vi "OS_Comm_to_Var_Binary.vi"(9 "Array 3":T1[](array[typedef]) {"Control" items=["Nul"=0, "Pulse On"=1, "Pulse Off"=2, "Latch On"=3, "Latch Off"=4, "Close"=65, "Trip"=129]}) -> ()   [LabVIEW 2016, in "DNP3_Outstation_Template.lvlib"]
uses:
  DNP3_Outstation_Template.lvlib
  <vilib>/DNP3/DNP3_Common/crob.ctl
  <vilib>/DNP3/DNP3_Common/crob_ctrl.ctl
  <vilib>/Utility/file.llb/Read Delimited Spreadsheet (string).vi
  <vilib>/DNP3/DNP3_Common.lvlib
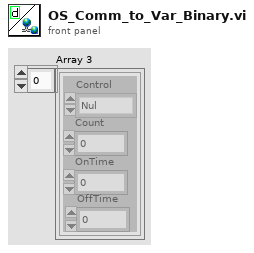
[diagram p1: front panel]
types:
  T1 = typedef "DNP3_Common.lvlib/crob.ctl" = cluster{"OnTime":u32, "Count":u8, "OffTime":u32, "Control":T2}
  T2 = typedef "DNP3_Common.lvlib/crob_ctrl.ctl" = u8
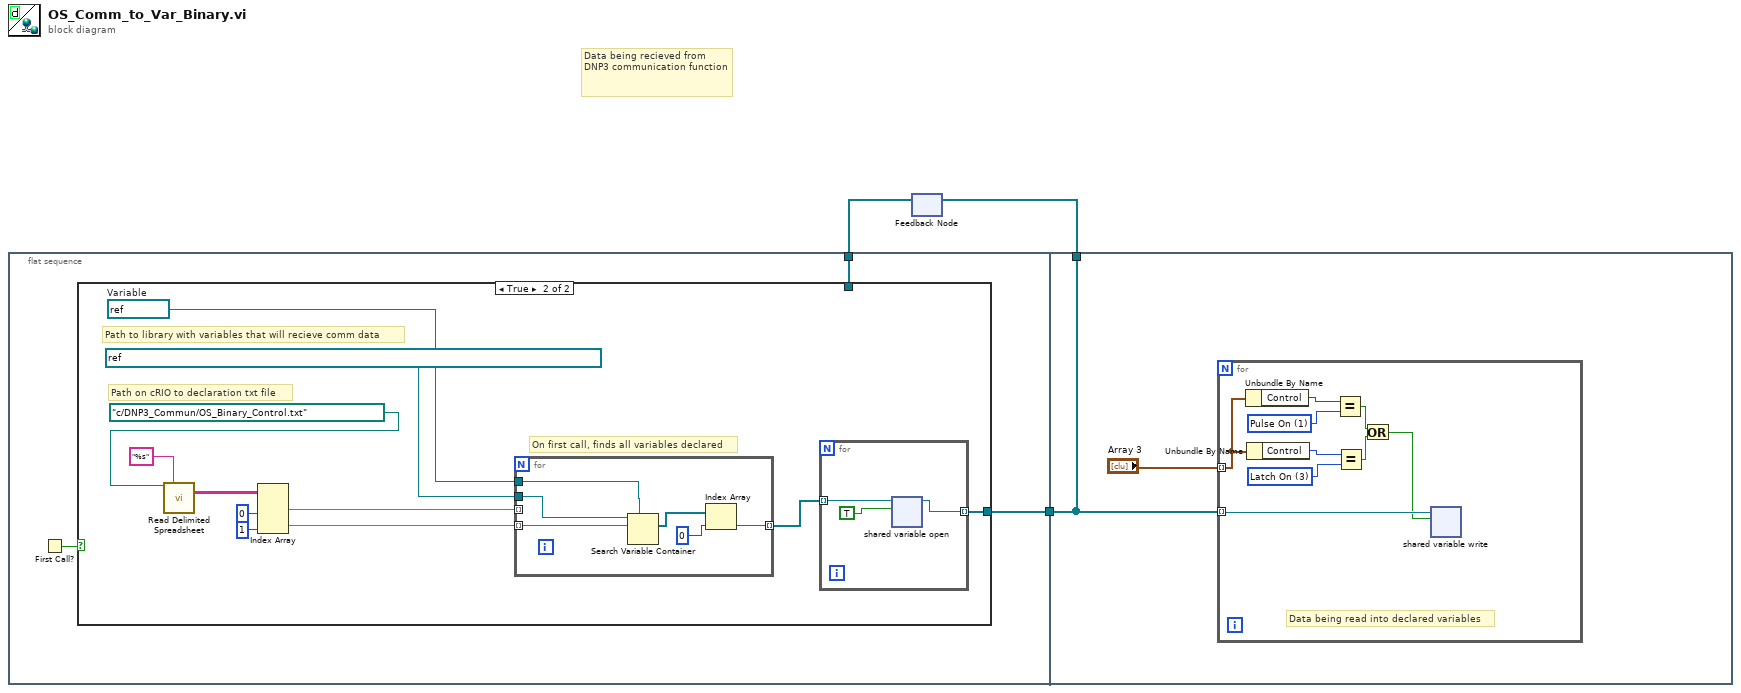
[diagram p0: block diagram]
diagram:
  # "Data being recieved from DNP3 communication function"
  n1 = flat-sequence {
    tunnel: [w5] -> w3
    tunnel: w1 -> [w4]
    tunnel: w3 -> [w28]
    tunnel: [w28] -> w2
    frame #0 {
      n2 = First Call?() -> (First Call?: T/F=w6:bool)
      n3 = case shown="True" w6 {
        tunnel: [w7 w8] -> w5
        tunnel: w4 -> [w7 _]
        frame False {
        }
        frame True {
          w10 = refnum<k21> refnum  # Variable
          # "On first call, finds all variables declared"
          # "Path on cRIO to declaration txt file"
          # "Path to library with variables that will recieve comm data"
          n4 = call-poly <vilib>:"Read Delimited Spreadsheet.vi"("file path (dialog if empty)"=path "c:/DNP3_Commun/OS_Binary_Control.txt" ("file path (use dialog)"), "format (%s)"="%s") -> ("all rows"=w14:string[][])  [unwired: 8 in, 5 out]
          n5 = Index Array(array=w14, index (col) #1=0 ("disabled index (col)"), index (col) #2=1 ("index (col)")) -> (element #1=w17:string[], element #2=w18:string[])  [unwired: 2 in]
          n6 = for {
            tunnel: w10 -> [w25]
            tunnel: refnum<k21> "ni.var.psp://lc1 (bess)/DNP3_Outstation_Template/OS_Data_Variables/OS_Binary_Control" ("container refnum in") -> [w24]
            tunnel: w17 -> [_] mode=indexing
            tunnel: w18 -> [w23] mode=indexing
            tunnel: [w22] -> w9 mode=indexing
            n7 = Search Variable Container(7:w25, 10:w23, 11:w24) -> (2:w27:refnum<k21>[])  [unwired: 3 in, 2 out]
            n8 = Index Array(array=w27, index=0) -> (element=w22:refnum<k21>)
          }
          n9 = for {
            tunnel: w9 -> [w20] mode=indexing
            tunnel: [w19] -> w8 mode=indexing
            n10 = shared-variable-open(w20, TRUE) -> (w19:refnum<k21>)  [unwired: 2 in, 1 out]
          }
        }
      }
    }
    frame #1 {
      n11 = for {
        tunnel: "Array 3" -> [w33] mode=indexing
        tunnel: w28 -> [w36] mode=indexing
        w35 = T2 1 items=["Nul"=0, "Pulse On"=1, "Pulse Off"=2, "Latch On"=3, "Latch Off"=4, "Close"=65, "Trip"=129] ("x")
        w37 = T2 3 items=["Nul"=0, "Pulse On"=1, "Pulse Off"=2, "Latch On"=3, "Latch Off"=4, "Close"=65, "Trip"=129] ("x")
        # "Data being read into declared variables"
        n12 = Unbundle By Name(w33) -> ("Control"=w34:T2)
        n13 = Unbundle By Name(w33) -> ("Control"=w38:T2)
        n14 = Equal?(x=w34, y=w35) -> (x = y?=w31:bool)
        n15 = Equal?(x=w38, y=w37) -> (x = y?=w32:bool)
        n16 = Or(x=w31, y=w32) -> (x .or. y?=w30:bool)
        n17 = shared-variable-write(w36, w30) -> ()  [unwired: 1 in, 2 out]
      }
    }
  }
  n18 = feedback-in #1(w2) -> ()
  n19 = feedback #1() -> (w1:refnum<k21>[])  [unwired: 1 in]
